vi "Data Acq Control.vi"(0 "Data Acquisition":T2=enum."NML Data Acquisition-New.vi", 1 "command text in":string[](array[string])) -> ()   [LabVIEW 2020]
uses:
  Ctl/Data Acquisition System.ctl
panel:
  out "error out 2":errorcluster
  out "New/Stop File":T1(ring)
  out "error out":errorcluster
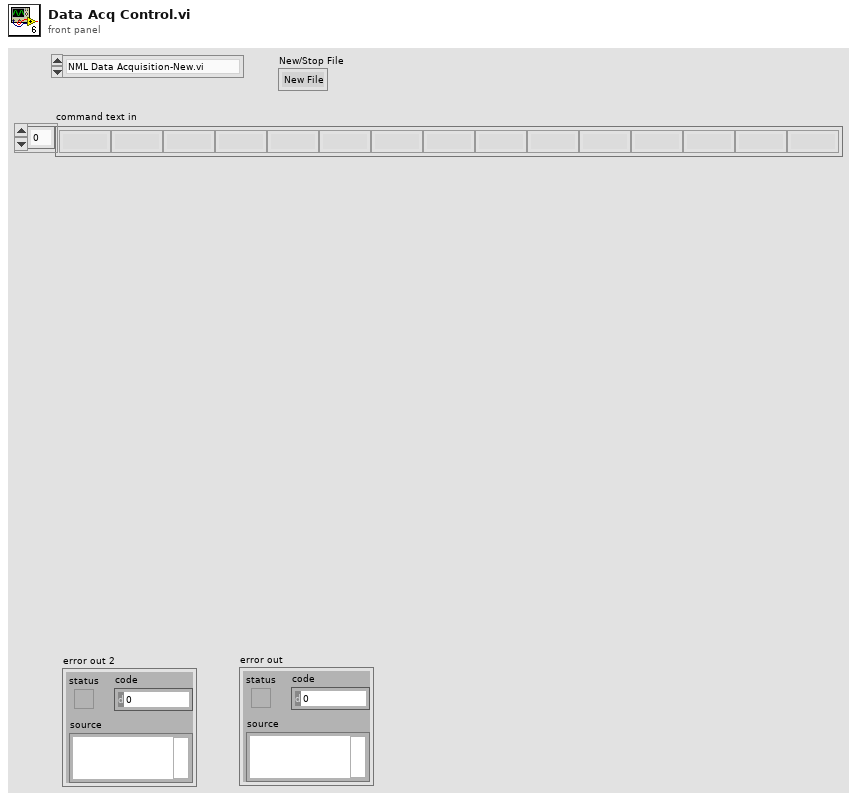
[diagram p1: front panel]
types:
  T1 = enum32{"New File", "Stop FIle", "Test", "Run", "Pause"}
  T2 = typedef "Data Acquisition System.ctl" = enum16{"NML Data Acquisition-old.vi", "NML Data Acquisition-New.vi"}
  T3 = typedef "Data Acq.ctl" = cluster{"New/Stop File":enum32{"New File", "Stop FIle", "Test", "Run", "Pause"}, "Comments Option":bool, "Comments":string, "extra wait":i32}
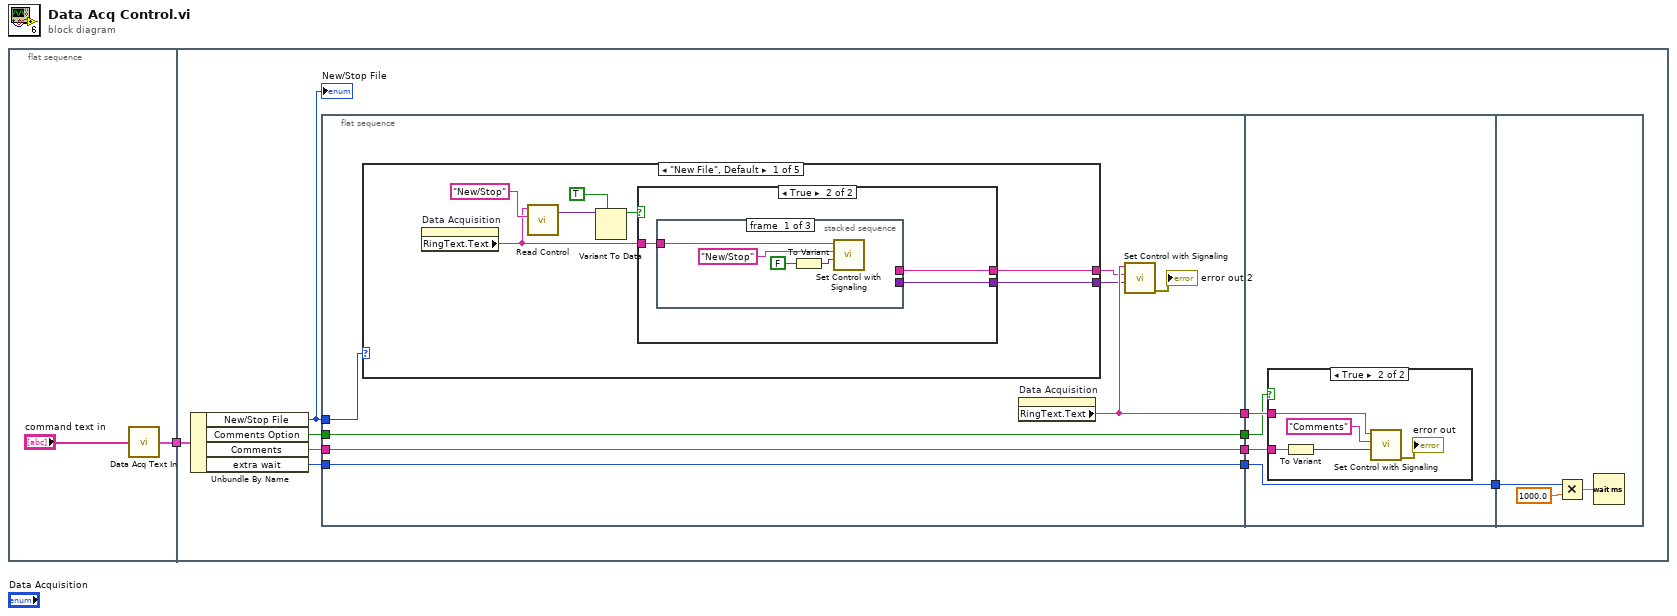
[diagram p0: block diagram]
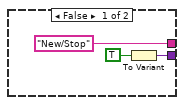
[diagram p2: hidden frame]
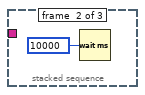
[diagram p3: hidden frame]
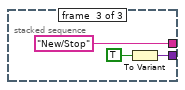
[diagram p4: hidden frame]
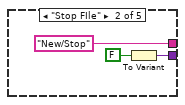
[diagram p5: hidden frame]
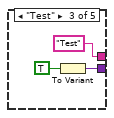
[diagram p6: hidden frame]
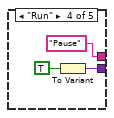
[diagram p7: hidden frame]
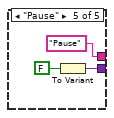
[diagram p8: hidden frame]
diagram:
  n1 = flat-sequence {
    tunnel: [w2] -> w1
    tunnel: w1 -> [w4]
    frame #0 {
      n2 = call "Data Acq Text In.vi"("command text in"="command text in") -> ("Data Acq"=w2:T3)
    }
    frame #1 {
      n3 = Unbundle By Name(w4) -> ("New/Stop File"=w7:T1, "Comments Option"=w8:bool, "Comments"=w6:string, "extra wait"=w5:i32)
      "New/Stop File" <- w7
      n4 = flat-sequence {
        tunnel: [w21] -> w13
        tunnel: [w20] -> w12
        tunnel: w8 -> [w20]
        tunnel: w7 -> [w19]
        tunnel: [w16] -> w11
        tunnel: w6 -> [w16]
        tunnel: w5 -> [w14]
        tunnel: [w14] -> w10
        tunnel: w13 -> [w58]
        tunnel: w12 -> [w57]
        tunnel: w11 -> [w56]
        tunnel: w10 -> [w55]
        tunnel: [w55] -> w9
        tunnel: w9 -> [w65]
        frame #0 {
          n5 = case shown="\"New File\", Default" w19 {
            tunnel: [w28 "New/Stop" ("Control Name") "Test" "Pause" "Pause"] -> w18
            tunnel: [w27 w43 w46 w50 w52] -> w17
            frame "New File", Default {
              n6 = property on="Data Acquisition" class="Enum (strict)"() -> ("RingText.Text"=w22:string)  [unwired: 2 in, 2 out]
              n7 = call "Read Control.vi"("VI Name"=w22, "Control Name"="New/Stop") -> ("Value"=w24:variant)  [unwired: 3 in, 1 out]
              n8 = Variant To Data(type=TRUE, Variant=w24) -> (data=w23:bool)  [unwired: 1 in, 1 out]
              n9 = case shown="True" w23 {
                tunnel: ["New/Stop" ("Control Name") w33] -> w28
                tunnel: [w29 w32] -> w27
                tunnel: w22 -> [_ w34]
                frame False {
                  n10 = To Variant(anything=TRUE) -> (Variant=w29:variant)
                }
                frame True {
                  n11 = stacked-sequence {
                    tunnel: w34 -> [w37 _ _]
                    tunnel: [_ _ "New/Stop" ("Control Name")] -> w33
                    tunnel: [_ _ w40] -> w32
                    frame #0 {
                      n12 = To Variant(anything=FALSE) -> (Variant=w35:variant)
                      n13 = call "Set Control with Signaling.vi"("Value"=w35, "Control Name"="New/Stop", "VI Name"=w37) -> ()  [unwired: 8 in, 1 out]
                    }
                    frame #1 {
                      n14 = Wait (ms)(milliseconds to wait=u32 10000) -> ()  [unwired: 1 out]
                    }
                    frame #2 {
                      n15 = To Variant(anything=TRUE) -> (Variant=w40:variant)
                    }
                  }
                }
              }
            }
            frame "Stop FIle" {
              n16 = To Variant(anything=FALSE) -> (Variant=w43:variant)
            }
            frame "Test" {
              n17 = To Variant(anything=TRUE) -> (Variant=w46:variant)
            }
            frame "Run" {
              n18 = To Variant(anything=TRUE) -> (Variant=w50:variant)
            }
            frame "Pause" {
              n19 = To Variant(anything=FALSE) -> (Variant=w52:variant)
            }
          }
          n20 = property on="Data Acquisition" class="Enum (strict)"() -> ("RingText.Text"=w21:string)  [unwired: 2 in, 2 out]
          n21 = call "Set Control with Signaling.vi"("Value"=w17, "Control Name"=w18, "VI Name"=w21) -> ("error out"=→"error out 2":errorcluster)  [unwired: 8 in]
        }
        frame #1 {
          n22 = case shown="True" w57 {
            tunnel: w58 -> [_ w62]
            tunnel: w56 -> [_ w60]
            frame False {
            }
            frame True {
              n23 = To Variant(anything=w60) -> (Variant=w63:variant)
              n24 = call "Set Control with Signaling.vi"("Value"=w63, "Control Name"="Comments", "VI Name"=w62) -> ("error out"=→"error out":errorcluster)  [unwired: 8 in]
            }
          }
        }
        frame #2 {
          n25 = Multiply(x=w65, y=1000.0) -> (x*y=w64:dbl)
          n26 = Wait (ms)(milliseconds to wait=w64) -> ()  [unwired: 1 out]
        }
      }
    }
  }
